vi "Six Motors Final.vi"() -> ()   [LabVIEW 2013]
uses:
  <vilib>/Analysis/Matrix/Datatypes/RealMatrix.ctl
  <vilib>/picture/3D Picture Control/Object/Create Object (drawable).vi
  <vilib>/picture/3D Picture Control/Object/Add Object (reference).vi
  <vilib>/Instr/_visa.llb/VISA Configure Serial Port (Instr).vi
  <vilib>/picture/3D Picture Control/NI_3D Picture Control.lvlib
  <vilib>/Analysis/Matrix/NI_Matrix.lvlib
panel:
  in  "Initial Values":bool
  out "x+y":dbl
  in  "Shoulder Angle":dbl=130.0
  in  "Pitch Exten":dbl
  in  "Elbow Angle":dbl=-130.0
  out "Input Palettes":string
  in  "Speed_PWM":i32(knob)=255 min=0 max=255 scale=0.0..255.0
  in  "Hard Home":bool
  in  "Pitch Closure":dbl(slide) min=0.0 max=130.0 scale=0.0..100.0
  out "FINAL TRANSFORMATION MATRIX":T1 format="%#.7f"
  in  "Base Angle":dbl
  in  "Pitch Roll":dbl
  in  "?":enum32{"Main Control", "Simulator"}(tab)
  out "Pitch Closure at Angle":i32
  out "Pitch Roll at Angle":i32
  out "Pitch Stretch at Angle":i32
  out "Elbow at Angle":i32
  out "Shoulder at Angle":i32
  out "Base at Angle":i16
  out "Position Palettes":string
  out "Error Palettes":string
  out "A Error":i32
  out "B Error":i32
  out "C Error":i32
  out "D Error":i32
  out "E Error":i32
  out "F Error":i32
  out "Serial Palettes":string
  out "Read Count":u32
  out "Write Count":u32
  in  "Home Position":bool
  out "Rhino Simulator":refnum<vi>(3d-picture)
  in  "Rhino Color":u32(colorbox)=11776947
  in  "Axis Color":u32(colorbox)
  in  "BackGround Color":u32(colorbox)=16777238
  in  "Alpha Value":dbl(slide)=0.47783251231527096 scale=0.0..1.0
  out "3D Picture 2":refnum<vi>(3d-picture)
  in  "STOP":bool
  in  "START":bool
  # "Close"
  # "Open"
  # "------------------------------------------------------- INSTRUCTIONS TO USE -------------------------------------------------------\n1 - This is a Rhino Simulator \n2 - Run the code and first select the Axis Color, Rhino Color , Background Color, Alpha Value and Object's Position w.r.t Rhino base\n3 - Press the Start Button. (At this point, you should be seeing a red cube, a rhino simulator and two axes, one moving and on non-moving).\n4 - Now change the angles of each joints (named with respect to the motors attached to them)\n5 - Get the values of angles which will eventually make the Rhino End Effector to move to the cubic object.\n6 - Now put these values in the orignal code and have fun! :) \n\nNote: At any point after pressing the Start button if either want to change the colors or object position, you will have to STOP the code and Run again."
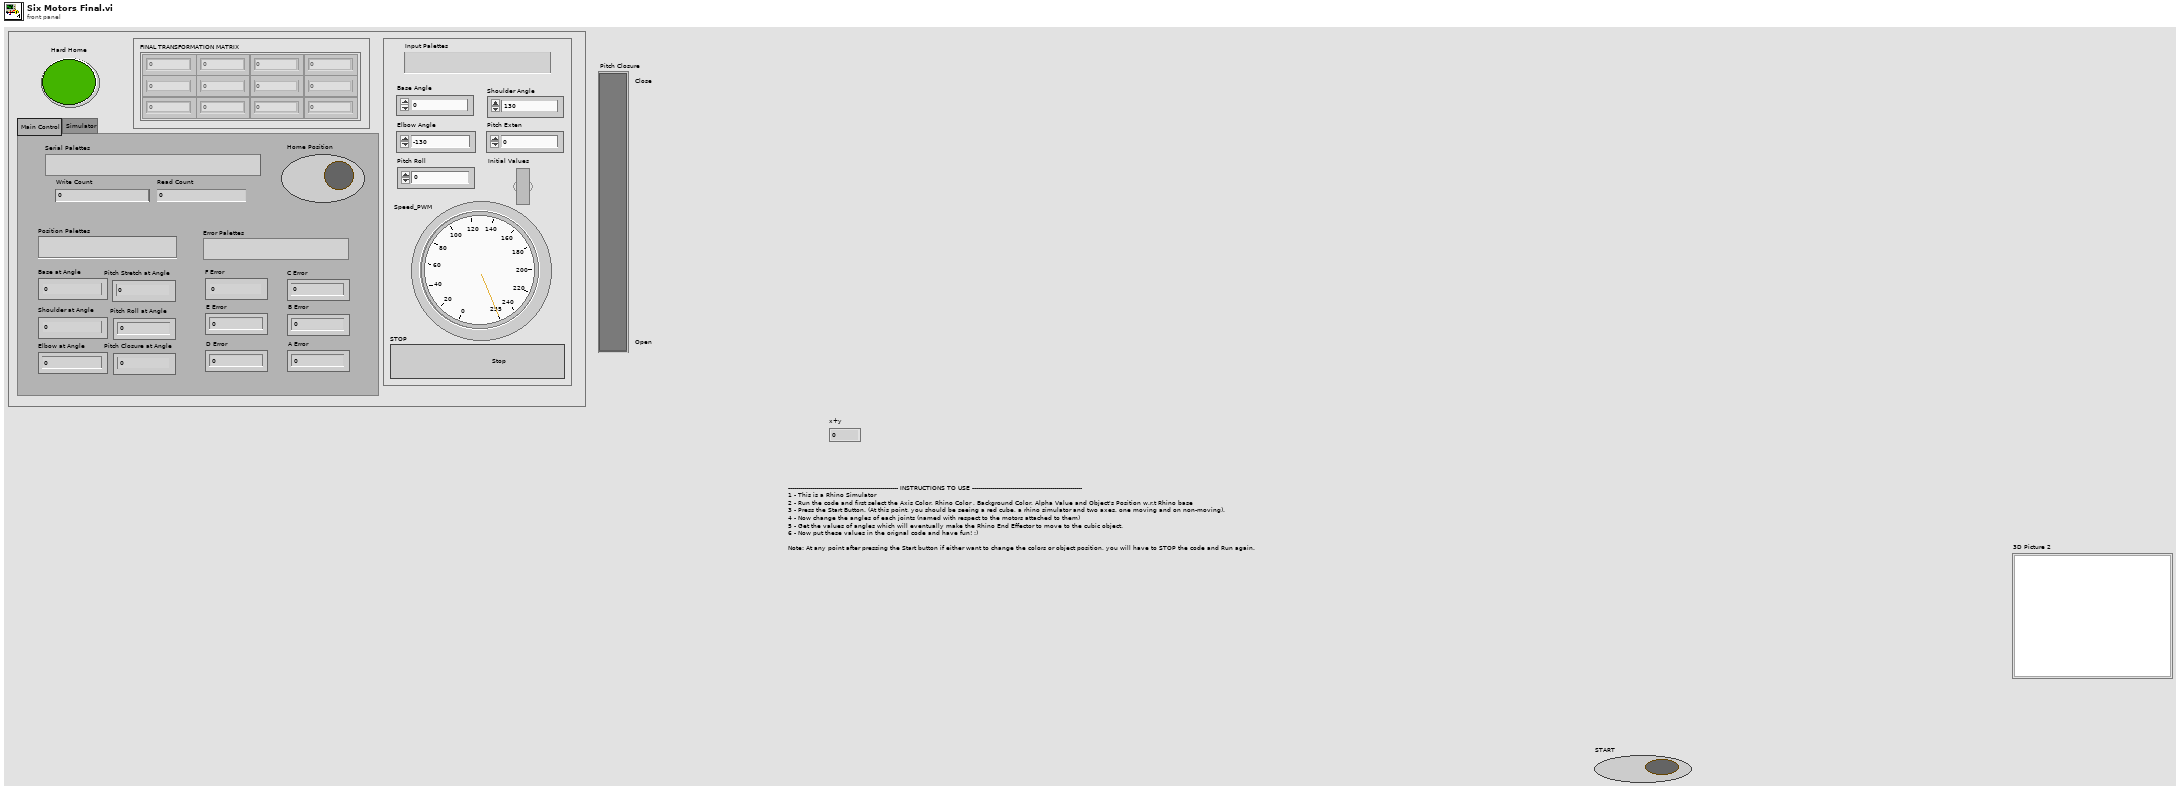
[diagram p1: front panel]
types:
  T1 = typedef "NI_Matrix.lvlib/RealMatrix.ctl" = dbl[][]
  T2 = cluster{"Red":sgl, "Green":sgl, "Blue":sgl, "Alpha":sgl}
  T3 = enum8{"Enabled", "Disabled", "Disabled and Grayed Out"}
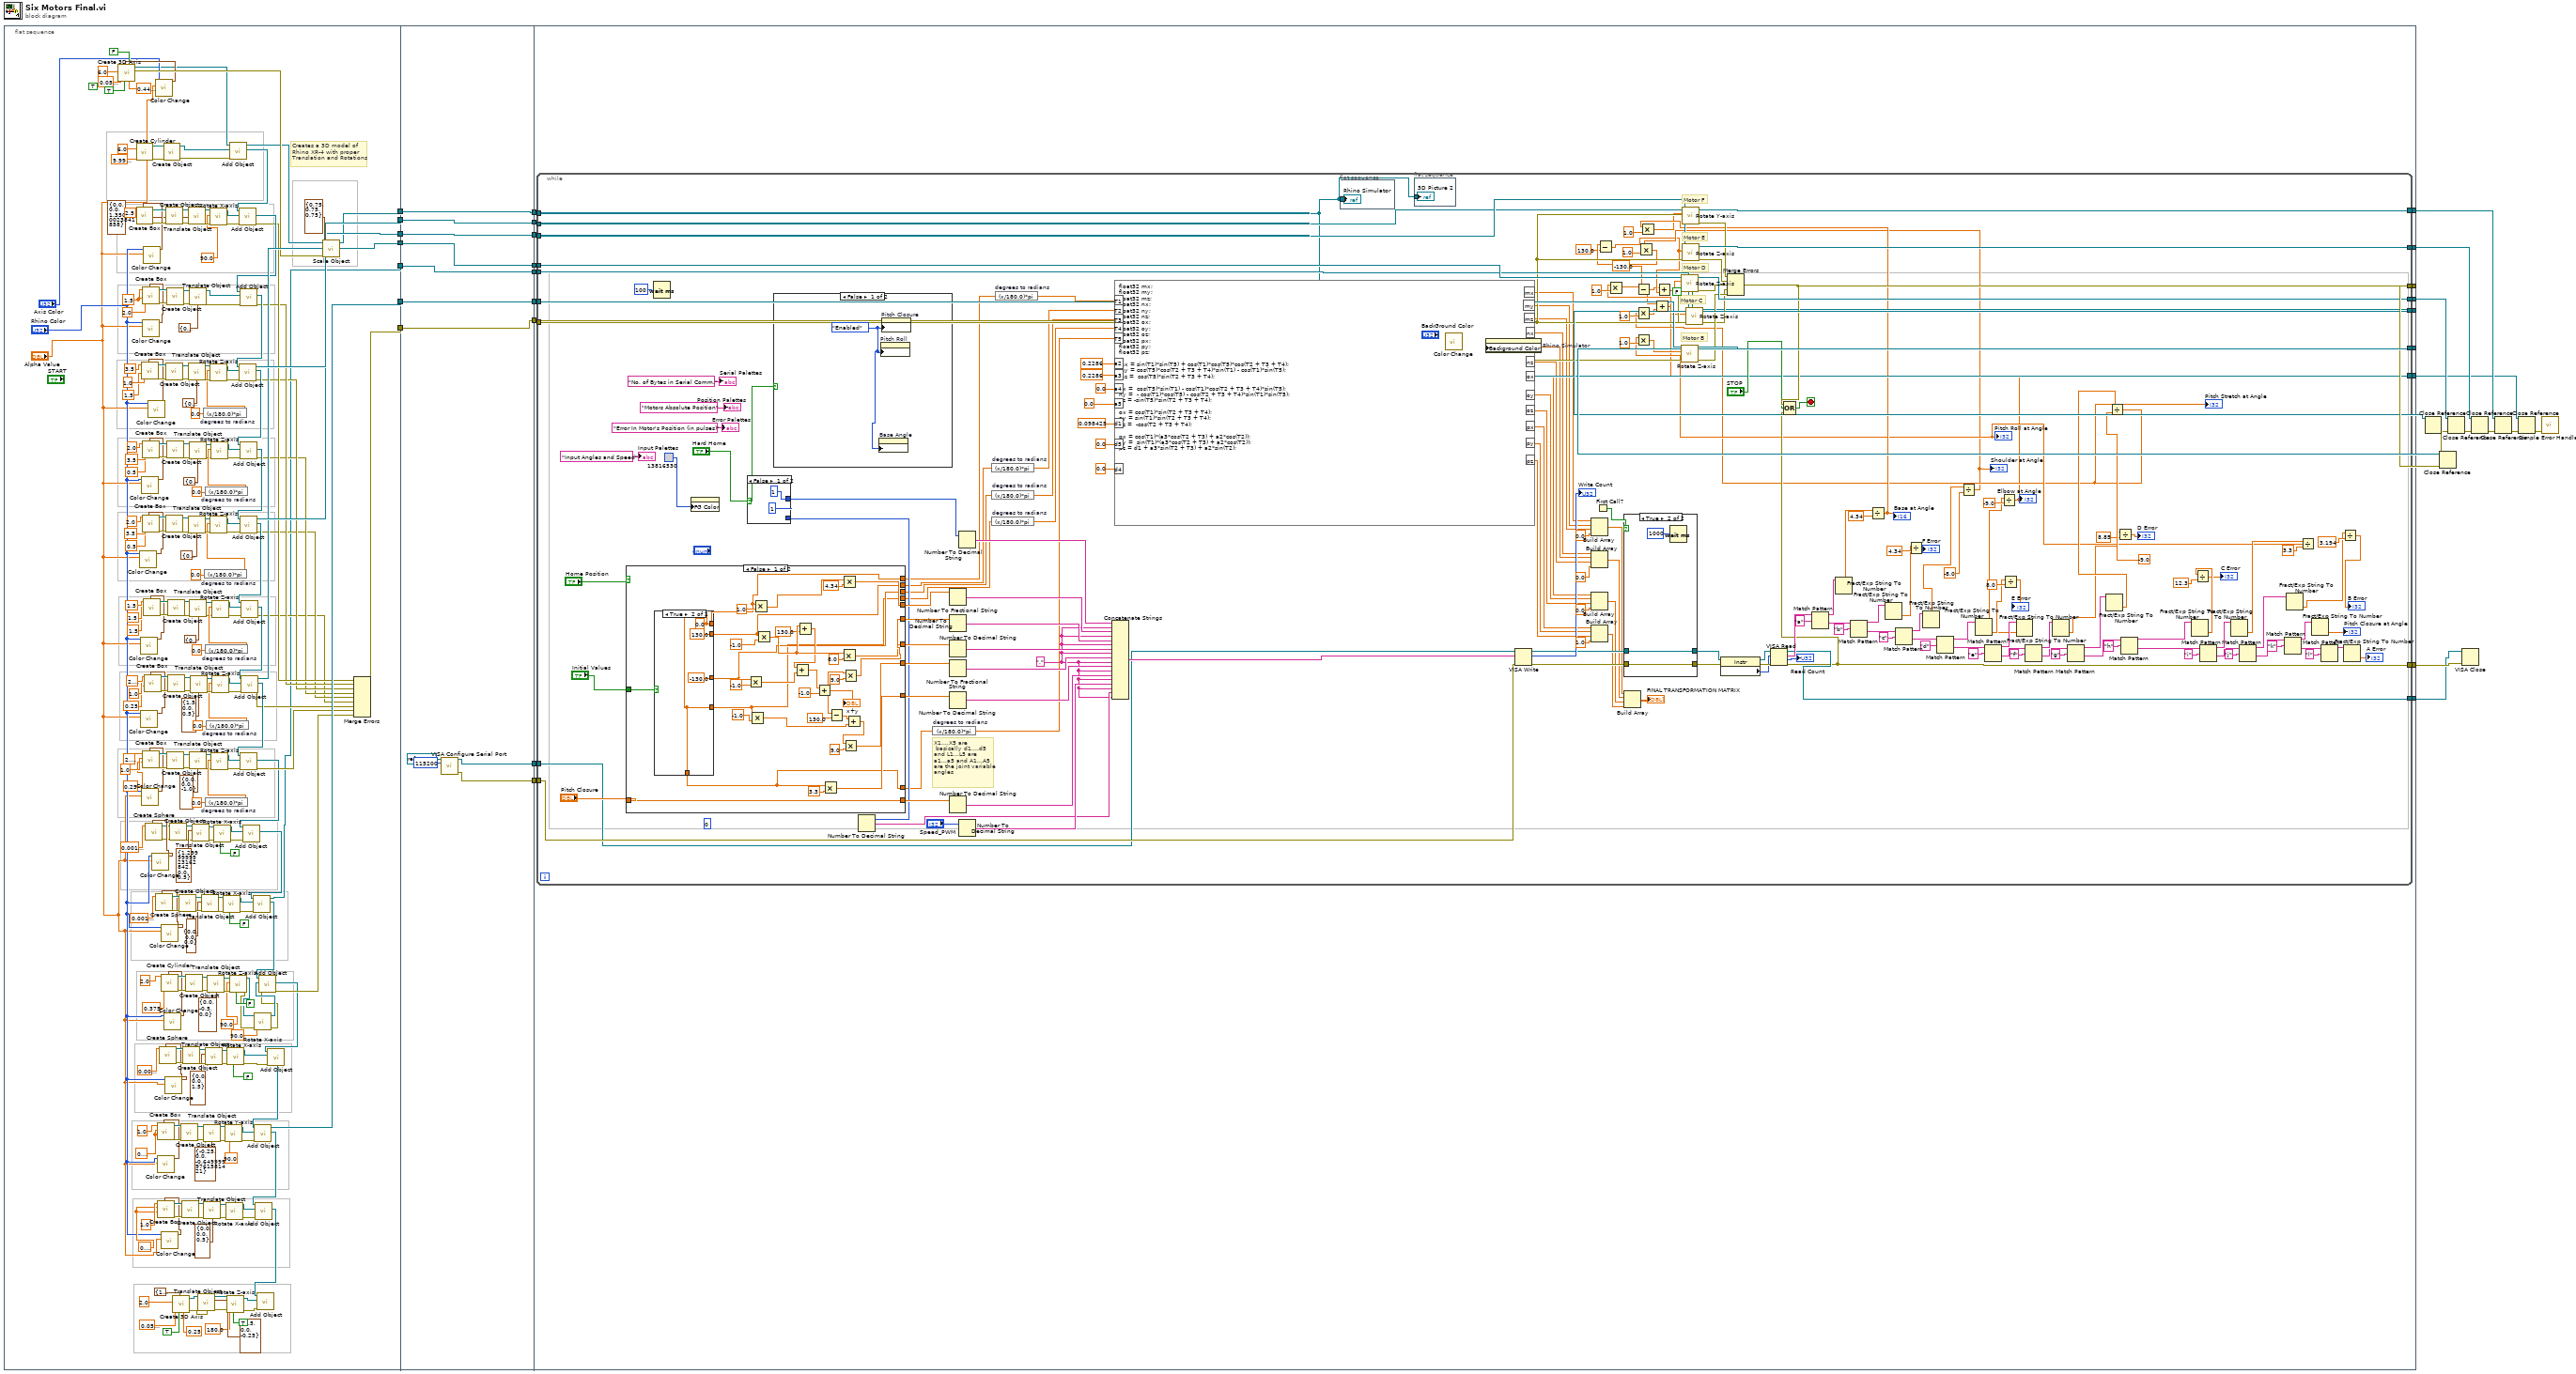
[diagram p0: block diagram]
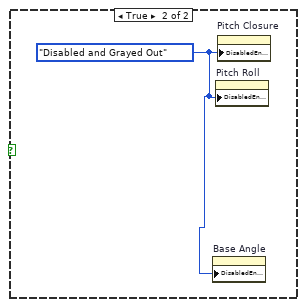
[diagram p2: hidden frame]
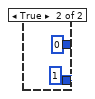
[diagram p3: hidden frame]
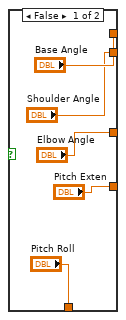
[diagram p4: hidden frame]
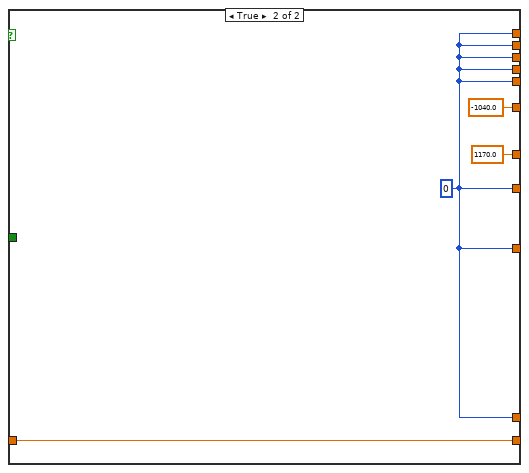
[diagram p5: hidden frame]
diagram:
  n1 = flat-sequence {
    tunnel: [w95] -> w31
    tunnel: [w285] -> w30
    tunnel: [w284] -> w29
    tunnel: [w283] -> w28
    tunnel: [w282] -> w27
    tunnel: [w38] -> w26
    tunnel: [w281] -> w25
    tunnel: [w296] -> w24
    tunnel: [w292] -> w23
    tunnel: [w290] -> w22
    tunnel: w31 -> [w296]
    tunnel: w30 -> [w295]
    tunnel: [w295] -> w21
    tunnel: w29 -> [w294]
    tunnel: [w294] -> w20
    tunnel: w28 -> [w293]
    tunnel: [w293] -> w19
    tunnel: w27 -> [w292]
    tunnel: w26 -> [w291]
    tunnel: [w291] -> w18
    tunnel: w25 -> [w290]
    tunnel: [w289] -> w4
    tunnel: [w288] -> w3
    tunnel: w24 -> [w314]
    tunnel: w23 -> [w310]
    tunnel: w22 -> [w311]
    tunnel: [w307] -> w13
    tunnel: [w306] -> w12
    tunnel: [w305] -> w11
    tunnel: [w304] -> w10
    tunnel: [w303] -> w9
    tunnel: [w302] -> w8
    tunnel: [w301] -> w6
    tunnel: w21 -> [w308]
    tunnel: w20 -> [w309]
    tunnel: w19 -> [w313]
    tunnel: w18 -> [w312]
    tunnel: w4 -> [w300]
    tunnel: w3 -> [w299]
    tunnel: [w298] -> w2
    tunnel: [w297] -> w1
    frame #0 {
      (unwired) TRUE ("Axis label?")
      w125 = sgl 0.1 ("Length Y")
      w127 = sgl 0.1 ("Length Y")
      w189 = sgl 1.5 ("Length X")
      w279 = sgl 2.5 ("Length X")
      # "Creates a 3D model of \nRhino XR-4 with proper \nTranslation and Rotations"
      n2 = call <vilib>:"Create Cylinder.vi"("Radius"=sgl 6.0, "Height"=sgl 0.0001) -> ("error out"=w77:errorcluster, "New Cylinder Refnum"=w78:refnum<vi>)  [unwired: 8 in]
      n3 = call <vilib>:"Color Change.vi"("Alpha"="Alpha Value", "Color"="Rhino Color") -> ("RGBA"=w115:cluster{"R":sgl, "G":sgl, "B":sgl, "A":sgl})  [unwired: 9 in]
      n4 = call <vilib>:"Color Change.vi"("Alpha"="Alpha Value", "Color"="Rhino Color") -> ("RGBA"=w116:cluster{"R":sgl, "G":sgl, "B":sgl, "A":sgl})  [unwired: 9 in]
      n5 = call <vilib>:"Color Change.vi"("Alpha"="Alpha Value", "Color"="Rhino Color") -> ("RGBA"=w117:cluster{"R":sgl, "G":sgl, "B":sgl, "A":sgl})  [unwired: 9 in]
      n6 = call <vilib>:"Color Change.vi"("Alpha"="Alpha Value", "Color"="Rhino Color") -> ("RGBA"=w113:cluster{"R":sgl, "G":sgl, "B":sgl, "A":sgl})  [unwired: 9 in]
      n7 = call <vilib>:"Color Change.vi"("Alpha"="Alpha Value", "Color"="Rhino Color") -> ("RGBA"=w118:cluster{"R":sgl, "G":sgl, "B":sgl, "A":sgl})  [unwired: 9 in]
      n8 = call <vilib>:"Create Box.vi"("Color"=w115, "Length Z"=sgl 0.5, "Length Y"=sgl 3.5, "Length X"=sgl 2.0) -> ("error out"=w234:errorcluster, "New Box Refnum"=w240:refnum<vi>)  [unwired: 6 in]
      n9 = call <vilib>:"Color Change.vi"("Alpha"="Alpha Value", "Color"="Rhino Color") -> ("RGBA"=w112:cluster{"R":sgl, "G":sgl, "B":sgl, "A":sgl})  [unwired: 9 in]
      n10 = call <vilib>:"Create Box.vi"("Color"=w112, "Length Z"=w189, "Length Y"=sgl 2.0, "Length X"=w189) -> ("error out"=w266:errorcluster, "New Box Refnum"=w263:refnum<vi>)  [unwired: 6 in]
      n11 = call <vilib>:"Create Box.vi"("Color"=w113, "Length Z"=sgl 0.5, "Length Y"=sgl 3.5, "Length X"=sgl 2.0) -> ("error out"=w247:errorcluster, "New Box Refnum"=w241:refnum<vi>)  [unwired: 6 in]
      n12 = call <vilib>:"Create Box.vi"("Color"=w118, "Length Z"=sgl 0.25 ("Length X"), "Length Y"=sgl 1.0 ("Length X"), "Length X"=sgl 2.7) -> ("error out"=w204:errorcluster, "New Box Refnum"=w198:refnum<vi>)  [unwired: 6 in]
      n13 = call <vilib>:"Color Change.vi"("Alpha"="Alpha Value", "Color"="Rhino Color") -> ("RGBA"=w123:cluster{"R":sgl, "G":sgl, "B":sgl, "A":sgl})  [unwired: 9 in]
      n14 = call <vilib>:"Create Box.vi"("Color"=w123, "Length Z"=w279, "Length Y"=w279, "Length X"=w279) -> ("error out"=w269:errorcluster, "New Box Refnum"=w280:refnum<vi>)  [unwired: 6 in]
      n15 = call <vilib>:"Create Box.vi"("Color"=w116, "Length Z"=sgl 1.5 ("Length X"), "Length Y"=sgl 1.5 ("Length X"), "Length X"=sgl 1.5) -> ("error out"=w226:errorcluster, "New Box Refnum"=w220:refnum<vi>)  [unwired: 6 in]
      n16 = call <vilib>:"Create Box.vi"("Color"=w117, "Length Z"=sgl 0.25 ("Length X"), "Length Y"=sgl 1.0 ("Length X"), "Length X"=sgl 2.7) -> ("error out"=w213:errorcluster, "New Box Refnum"=w219:refnum<vi>)  [unwired: 6 in]
      n17 = call <vilib>:"Color Change.vi"("Alpha"="Alpha Value", "Color"="Rhino Color") -> ("RGBA"=w114:cluster{"R":sgl, "G":sgl, "B":sgl, "A":sgl})  [unwired: 9 in]
      n18 = call <vilib>:"Create Box.vi"("Color"=w114, "Length Z"=sgl 1.5, "Length Y"=sgl 1.0, "Length X"=sgl 3.5) -> ("error out"=w256:errorcluster, "New Box Refnum"=w262:refnum<vi>)  [unwired: 6 in]
      n19 = call <vilib>:"Color Change.vi"("Alpha"="Alpha Value", "Color"="Rhino Color") -> ("RGBA"=w67:cluster{"R":sgl, "G":sgl, "B":sgl, "A":sgl})  [unwired: 9 in]
      n20 = call <vilib>:"Create Sphere.vi"("Color"=w67, "Radius"=sgl 0.001 ("Length X")) -> ("error out"=w59:errorcluster, "New Sphere Refnum"=w65:refnum<vi>)  [unwired: 8 in]
      n21 = call <vilib>:"Color Change.vi"("Alpha"="Alpha Value", "Color"="Axis Color") -> ("RGBA"=w111:cluster{"R":sgl, "G":sgl, "B":sgl, "A":sgl})  [unwired: 9 in]
      n22 = call <vilib>:"Create 3D Axis.vi"("Character Size"=sgl 0.45, "Half plane?"=FALSE, "Axis label?"=TRUE, "Color"=w111, "Radius"=sgl 0.05, "Length"=sgl 6.0) -> ("error out"=w161:errorcluster, "New Object Refnum"=w75:refnum<vi>)  [unwired: 4 in]
      n23 = call <vilib>:"Color Change.vi"("Alpha"="Alpha Value", "Color"="Rhino Color") -> ("RGBA"=w120:cluster{"R":sgl, "G":sgl, "B":sgl, "A":sgl})  [unwired: 9 in]
      n24 = call <vilib>:"Create Box.vi"("Color"=w120, "Length Z"=w127, "Length Y"=w127, "Length X"=sgl 1.0) -> ("error out"=w145:errorcluster, "New Box Refnum"=w139:refnum<vi>)  [unwired: 6 in]
      n25 = call <vilib>:"Color Change.vi"("Alpha"="Alpha Value", "Color"="Rhino Color") -> ("RGBA"=w121:cluster{"R":sgl, "G":sgl, "B":sgl, "A":sgl})  [unwired: 9 in]
      n26 = call <vilib>:"Create Box.vi"("Color"=w121, "Length Z"=w125, "Length Y"=w125, "Length X"=sgl 1.0) -> ("error out"=w132:errorcluster, "New Box Refnum"=w138:refnum<vi>)  [unwired: 6 in]
      n27 = call <vilib>:"Color Change.vi"("Alpha"="Alpha Value", "Color"="Rhino Color") -> ("RGBA"=w43:cluster{"R":sgl, "G":sgl, "B":sgl, "A":sgl})  [unwired: 9 in]
      n28 = call <vilib>:"Create Sphere.vi"("Color"=w43, "Radius"=sgl 0.001 ("Length X")) -> ("error out"=w51:errorcluster, "New Sphere Refnum"=w45:refnum<vi>)  [unwired: 8 in]
      n29 = call-poly <vilib>:"Create Object.vi"("error in (no error)"=w77, "Geometry"=w78) -> ("error out"=w33:errorcluster, "Scene:New Object"=w34:refnum<vi>)  [unwired: 8 in]
      n30 = call <vilib>:"Color Change.vi"("Alpha"="Alpha Value", "Color"="Rhino Color") -> ("RGBA"=w119:cluster{"R":sgl, "G":sgl, "B":sgl, "A":sgl})  [unwired: 9 in]
      n31 = call <vilib>:"Create Cylinder.vi"("Color"=w119, "Radius"=sgl 0.375, "Height"=sgl 2.0) -> ("error out"=w193:errorcluster, "New Cylinder Refnum"=w197:refnum<vi>)  [unwired: 7 in]
      n32 = call <vilib>:"Color Change.vi"("Alpha"="Alpha Value", "Color"="Rhino Color") -> ("RGBA"=w98:cluster{"R":sgl, "G":sgl, "B":sgl, "A":sgl})  [unwired: 9 in]
      n33 = call <vilib>:"Create Sphere.vi"("Color"=w98, "Radius"=sgl 0.01 ("Length X")) -> ("error out"=w106:errorcluster, "New Sphere Refnum"=w100:refnum<vi>)  [unwired: 8 in]
      n34 = call-poly <vilib>:"Create Object.vi"("error in (no error)"=w269, "Geometry"=w280) -> ("error out"=w270:errorcluster, "Scene:New Object"=w274:refnum<vi>)  [unwired: 8 in]
      n35 = call-poly <vilib>:"Create Object.vi"("error in (no error)"=w256, "Geometry"=w262) -> ("error out"=w257:errorcluster, "Scene:New Object"=w261:refnum<vi>)  [unwired: 8 in]
      n36 = call-poly <vilib>:"Create Object.vi"("error in (no error)"=w234, "Geometry"=w240) -> ("error out"=w235:errorcluster, "Scene:New Object"=w239:refnum<vi>)  [unwired: 8 in]
      n37 = call-poly <vilib>:"Create Object.vi"("error in (no error)"=w266, "Geometry"=w263) -> ("error out"=w265:errorcluster, "Scene:New Object"=w264:refnum<vi>)  [unwired: 8 in]
      n38 = call-poly <vilib>:"Create Object.vi"("error in (no error)"=w247, "Geometry"=w241) -> ("error out"=w246:errorcluster, "Scene:New Object"=w242:refnum<vi>)  [unwired: 8 in]
      n39 = call-poly <vilib>:"Create Object.vi"("error in (no error)"=w204, "Geometry"=w198) -> ("error out"=w203:errorcluster, "Scene:New Object"=w199:refnum<vi>)  [unwired: 8 in]
      n40 = call-poly <vilib>:"Create Object.vi"("error in (no error)"=w226, "Geometry"=w220) -> ("error out"=w225:errorcluster, "Scene:New Object"=w221:refnum<vi>)  [unwired: 8 in]
      n41 = call-poly <vilib>:"Create Object.vi"("error in (no error)"=w213, "Geometry"=w219) -> ("error out"=w214:errorcluster, "Scene:New Object"=w218:refnum<vi>)  [unwired: 8 in]
      n42 = call-poly <vilib>:"Create Object.vi"("error in (no error)"=w59, "Geometry"=w65) -> ("error out"=w60:errorcluster, "Scene:New Object"=w64:refnum<vi>)  [unwired: 8 in]
      n43 = call <vilib>:"Create 3D Axis.vi"("Character Size"=sgl 0.25, "Axis label?"=TRUE, "Color"=T2 {"Red"=1.0, "Green"=0.0, "Blue"=1.0, "Alpha"=1.0}, "Radius"=sgl 0.05, "Length"=sgl 2.0) -> ("error out"=w86:errorcluster, "New Object Refnum"=w87:refnum<vi>)  [unwired: 5 in]
      n44 = call-poly <vilib>:"Create Object.vi"("error in (no error)"=w51, "Geometry"=w45) -> ("error out"=w50:errorcluster, "Scene:New Object"=w46:refnum<vi>)  [unwired: 8 in]
      n45 = call-poly <vilib>:"Create Object.vi"("error in (no error)"=w145, "Geometry"=w139) -> ("error out"=w144:errorcluster, "Scene:New Object"=w140:refnum<vi>)  [unwired: 8 in]
      n46 = call-poly <vilib>:"Create Object.vi"("error in (no error)"=w132, "Geometry"=w138) -> ("error out"=w133:errorcluster, "Scene:New Object"=w137:refnum<vi>)  [unwired: 8 in]
      n47 = call-poly <vilib>:"Create Object.vi"("error in (no error)"=w106, "Geometry"=w100) -> ("error out"=w105:errorcluster, "Scene:New Object"=w101:refnum<vi>)  [unwired: 8 in]
      n48 = call-poly <vilib>:"Create Object.vi"("error in (no error)"=w193, "Geometry"=w197) -> ("error out"=w194:errorcluster, "Scene:New Object"=w196:refnum<vi>)  [unwired: 8 in]
      n49 = call <vilib>:"Translate Object.vi"("error in (no error)"=w270, "Translation"=cluster{"X":sgl, "Y":sgl, "Z":sgl} {"X"=0.0, "Y"=0.0, "Z"=1.35}, "Scene.Object In"=w274) -> ("error out"=w271:errorcluster, "Scene.Object Out"=w268:refnum<vi>)  [unwired: 7 in]
      n50 = call <vilib>:"Translate Object.vi"("error in (no error)"=w257, "Translation"=cluster{"X":sgl, "Y":sgl, "Z":sgl} {"X"=0.5, "Y"=1.0, "Z"=0.0}, "Scene.Object In"=w261) -> ("error out"=w258:errorcluster, "Scene.Object Out"=w255:refnum<vi>)  [unwired: 7 in]
      n51 = call <vilib>:"Translate Object.vi"("error in (no error)"=w235, "Translation"=cluster{"X":sgl, "Y":sgl, "Z":sgl} {"X"=0.0, "Y"=0.0, "Z"=-2.0}, "Scene.Object In"=w239) -> ("error out"=w236:errorcluster, "Scene.Object Out"=w233:refnum<vi>)  [unwired: 7 in]
      n52 = call <vilib>:"Translate Object.vi"("error in (no error)"=w265, "Translation"=cluster{"X":sgl, "Y":sgl, "Z":sgl} {"X"=0.0, "Y"=1.0, "Z"=0.0}, "Scene.Object In"=w264) -> ("error out"=w148:errorcluster, "Scene.Object Out"=w149:refnum<vi>)  [unwired: 7 in]
      n53 = call <vilib>:"Translate Object.vi"("error in (no error)"=w246, "Translation"=cluster{"X":sgl, "Y":sgl, "Z":sgl} {"X"=0.7, "Y"=1.3, "Z"=1.0}, "Scene.Object In"=w242) -> ("error out"=w245:errorcluster, "Scene.Object Out"=w248:refnum<vi>)  [unwired: 7 in]
      n54 = call <vilib>:"Translate Object.vi"("error in (no error)"=w203, "Translation"=cluster{"X":sgl, "Y":sgl, "Z":sgl} {"X"=0.0, "Y"=0.0, "Z"=-1.0}, "Scene.Object In"=w199) -> ("error out"=w202:errorcluster, "Scene.Object Out"=w205:refnum<vi>)  [unwired: 7 in]
      n55 = call <vilib>:"Translate Object.vi"("error in (no error)"=w225, "Translation"=cluster{"X":sgl, "Y":sgl, "Z":sgl} {"X"=0.0, "Y"=1.8, "Z"=1.0}, "Scene.Object In"=w221) -> ("error out"=w224:errorcluster, "Scene.Object Out"=w227:refnum<vi>)  [unwired: 7 in]
      n56 = call <vilib>:"Translate Object.vi"("error in (no error)"=w214, "Translation"=cluster{"X":sgl, "Y":sgl, "Z":sgl} {"X"=1.5, "Y"=0.0, "Z"=0.5}, "Scene.Object In"=w218) -> ("error out"=w215:errorcluster, "Scene.Object Out"=w212:refnum<vi>)  [unwired: 7 in]
      n57 = call <vilib>:"Translate Object.vi"("error in (no error)"=w60, "Translation"=cluster{"X":sgl, "Y":sgl, "Z":sgl} {"X"=1.3, "Y"=0.0, "Z"=0.5}, "Scene.Object In"=w64) -> ("error out"=w61:errorcluster, "Scene.Object Out"=w58:refnum<vi>)  [unwired: 7 in]
      n58 = call <vilib>:"Translate Object.vi"("error in (no error)"=w86, "Translation"=cluster{"X":sgl, "Y":sgl, "Z":sgl} {"X"=0.5, "Y"=0.0, "Z"=-0.25}, "Scene.Object In"=w87) -> ("error out"=w83:errorcluster, "Scene.Object Out"=w84:refnum<vi>)  [unwired: 7 in]
      n59 = call <vilib>:"Translate Object.vi"("error in (no error)"=w50, "Translation"=cluster{"X":sgl, "Y":sgl, "Z":sgl} {"X"=0.0, "Y"=0.0, "Z"=0.0}, "Scene.Object In"=w46) -> ("error out"=w49:errorcluster, "Scene.Object Out"=w52:refnum<vi>)  [unwired: 7 in]
      n60 = call <vilib>:"Translate Object.vi"("error in (no error)"=w144, "Translation"=cluster{"X":sgl, "Y":sgl, "Z":sgl} {"X"=-0.25, "Y"=0.0, "Z"=-0.65}, "Scene.Object In"=w140) -> ("error out"=w143:errorcluster, "Scene.Object Out"=w146:refnum<vi>)  [unwired: 7 in]
      n61 = expression code="(x/180.0)*pi" "degrees to radians"(0.0) -> (w253:dbl)
      n62 = call <vilib>:"Translate Object.vi"("error in (no error)"=w133, "Translation"=cluster{"X":sgl, "Y":sgl, "Z":sgl} {"X"=0.0, "Y"=0.0, "Z"=0.5}, "Scene.Object In"=w137) -> ("error out"=w134:errorcluster, "Scene.Object Out"=w131:refnum<vi>)  [unwired: 7 in]
      n63 = expression code="(x/180.0)*pi" "degrees to radians"(0.0) -> (w231:dbl)
      n64 = expression code="(x/180.0)*pi" "degrees to radians"(0.0) -> (w250:dbl)
      n65 = expression code="(x/180.0)*pi" "degrees to radians"(0.0) -> (w207:dbl)
      n66 = expression code="(x/180.0)*pi" "degrees to radians"(0.0) -> (w228:dbl)
      n67 = call <vilib>:"Translate Object.vi"("error in (no error)"=w105, "Translation"=cluster{"X":sgl, "Y":sgl, "Z":sgl} {"X"=0.0, "Y"=0.0, "Z"=1.5}, "Scene.Object In"=w101) -> ("error out"=w104:errorcluster, "Scene.Object Out"=w107:refnum<vi>)  [unwired: 7 in]
      n68 = expression code="(x/180.0)*pi" "degrees to radians"(0.0) -> (w210:dbl)
      n69 = call <vilib>:"Translate Object.vi"("error in (no error)"=w194, "Translation"=cluster{"X":sgl, "Y":sgl, "Z":sgl} {"X"=0.0, "Y"=-0.5, "Z"=0.0}, "Scene.Object In"=w196) -> ("error out"=w195:errorcluster, "Scene.Object Out"=w192:refnum<vi>)  [unwired: 7 in]
      n70 = call <vilib>:"Rotate X-axis.vi"("error in (no error)"=w271, "angle"=90.0, "Scene Object In"=w268) -> ("error out"=w273:errorcluster, "Scene Object Out"=w272:refnum<vi>)  [unwired: 7 in]
      n71 = call <vilib>:"Rotate Z-axis.vi"("error in (no error)"=w258, "angle"=w253, "Scene Object In"=w255) -> ("error out"=w260:errorcluster, "Scene Object Out"=w259:refnum<vi>)  [unwired: 7 in]
      n72 = call <vilib>:"Rotate Z-axis.vi"("error in (no error)"=w236, "angle"=w231, "Scene Object In"=w233) -> ("error out"=w238:errorcluster, "Scene Object Out"=w237:refnum<vi>)  [unwired: 7 in]
      n73 = call <vilib>:"Rotate Z-axis.vi"("error in (no error)"=w245, "angle"=w250, "Scene Object In"=w248) -> ("error out"=w243:errorcluster, "Scene Object Out"=w244:refnum<vi>)  [unwired: 7 in]
      n74 = call <vilib>:"Rotate Z-axis.vi"("error in (no error)"=w202, "angle"=w207, "Scene Object In"=w205) -> ("error out"=w200:errorcluster, "Scene Object Out"=w201:refnum<vi>)  [unwired: 7 in]
      n75 = call <vilib>:"Rotate Z-axis.vi"("error in (no error)"=w224, "angle"=w228, "Scene Object In"=w227) -> ("error out"=w222:errorcluster, "Scene Object Out"=w223:refnum<vi>)  [unwired: 7 in]
      n76 = call <vilib>:"Rotate Z-axis.vi"("error in (no error)"=w215, "angle"=w210, "Scene Object In"=w212) -> ("error out"=w217:errorcluster, "Scene Object Out"=w216:refnum<vi>)  [unwired: 7 in]
      n77 = call <vilib>:"Rotate X-axis.vi"("Relative?"=FALSE, "error in (no error)"=w61, "Scene Object In"=w58) -> ("error out"=w63:errorcluster, "Scene Object Out"=w62:refnum<vi>)  [unwired: 7 in]
      n78 = call <vilib>:"Rotate X-axis.vi"("Relative?"=FALSE, "error in (no error)"=w49, "Scene Object In"=w52) -> ("error out"=w47:errorcluster, "Scene Object Out"=w48:refnum<vi>)  [unwired: 7 in]
      n79 = call <vilib>:"Rotate Y-axis.vi"("error in (no error)"=w143, "angle"=90.0, "Scene Object In"=w146) -> ("error out"=w141:errorcluster, "Scene Object Out"=w142:refnum<vi>)  [unwired: 7 in]
      n80 = call <vilib>:"Rotate X-axis.vi"("error in (no error)"=w134, "Scene Object In"=w131) -> ("error out"=w136:errorcluster, "Scene Object Out"=w135:refnum<vi>)  [unwired: 8 in]
      n81 = call <vilib>:"Rotate Z-axis.vi"("Relative?"=TRUE, "error in (no error)"=w83, "angle"=sgl 180.0, "Scene Object In"=w84) -> ("error out"=w82:errorcluster, "Scene Object Out"=w81:refnum<vi>)  [unwired: 6 in]
      n82 = call <vilib>:"Rotate X-axis.vi"("Relative?"=FALSE, "error in (no error)"=w104, "Scene Object In"=w107) -> ("error out"=w102:errorcluster, "Scene Object Out"=w103:refnum<vi>)  [unwired: 7 in]
      n83 = call-poly <vilib>:"Add Object.vi"("error in (no error)"=w33, "New Object In"=w34, "Scene Object In"=w75) -> ("New Object Out"=w76:refnum<vi>, "Scene Object Out"=w74:refnum<vi>)  [unwired: 6 in, 1 out]
      n84 = call <vilib>:"Rotate Z-axis.vi"("Relative?"=FALSE, "error in (no error)"=w195, "angle"=90.0, "Scene Object In"=w192) -> ("error out"=w70:errorcluster, "Scene Object Out"=w72:refnum<vi>)  [unwired: 6 in]
      n85 = call-poly <vilib>:"Add Object.vi"("error in (no error)"=w273, "New Object In"=w272, "Scene Object In"=w76) -> ("error out"=w160:errorcluster, "New Object Out"=w169:refnum<vi>)  [unwired: 6 in, 1 out]
      n86 = call-poly <vilib>:"Add Object.vi"("error in (no error)"=w148, "New Object In"=w149, "Scene Object In"=w169) -> ("error out"=w159:errorcluster, "New Object Out"=w168:refnum<vi>)  [unwired: 6 in, 1 out]
      n87 = call-poly <vilib>:"Add Object.vi"("error in (no error)"=w260, "New Object In"=w259, "Scene Object In"=w168) -> ("error out"=w158:errorcluster, "New Object Out"=w167:refnum<vi>, "Scene Object Out"=w285:refnum<vi>)  [unwired: 6 in]
      n88 = call-poly <vilib>:"Add Object.vi"("error in (no error)"=w243, "New Object In"=w244, "Scene Object In"=w167) -> ("error out"=w157:errorcluster, "New Object Out"=w166:refnum<vi>)  [unwired: 6 in, 1 out]
      n89 = call-poly <vilib>:"Add Object.vi"("error in (no error)"=w238, "New Object In"=w237, "Scene Object In"=w166) -> ("error out"=w156:errorcluster, "New Object Out"=w165:refnum<vi>, "Scene Object Out"=w284:refnum<vi>)  [unwired: 6 in]
      n90 = call-poly <vilib>:"Add Object.vi"("error in (no error)"=w222, "New Object In"=w223, "Scene Object In"=w165) -> ("error out"=w155:errorcluster, "New Object Out"=w164:refnum<vi>)  [unwired: 6 in, 1 out]
      n91 = call-poly <vilib>:"Add Object.vi"("error in (no error)"=w217, "New Object In"=w216, "Scene Object In"=w164) -> ("error out"=w154:errorcluster, "New Object Out"=w163:refnum<vi>, "Scene Object Out"=w283:refnum<vi>)  [unwired: 6 in]
      n92 = call-poly <vilib>:"Add Object.vi"("error in (no error)"=w200, "New Object In"=w201, "Scene Object In"=w163) -> ("error out"=w153:errorcluster, "New Object Out"=w55:refnum<vi>)  [unwired: 6 in, 1 out]
      n93 = call-poly <vilib>:"Add Object.vi"("error in (no error)"=w63, "New Object In"=w62, "Scene Object In"=w55) -> ("New Object Out"=w42:refnum<vi>)  [unwired: 6 in, 2 out]
      n94 = call-poly <vilib>:"Add Object.vi"("error in (no error)"=w47, "New Object In"=w48, "Scene Object In"=w42) -> ("New Object Out"=w41:refnum<vi>, "Scene Object Out"=w38:refnum<vi>)  [unwired: 6 in, 1 out]
      n95 = call <vilib>:"Rotate X-axis.vi"("error in (no error)"=w70, "angle"=90.0, "Scene Object In"=w72) -> ("error out"=w69:errorcluster, "Scene Object Out"=w71:refnum<vi>)  [unwired: 7 in]
      n96 = call-poly <vilib>:"Add Object.vi"("error in (no error)"=w69, "New Object In"=w71, "Scene Object In"=w41) -> ("error out"=w152:errorcluster, "New Object Out"=w32:refnum<vi>)  [unwired: 6 in, 1 out]
      n97 = call-poly <vilib>:"Add Object.vi"("error in (no error)"=w102, "New Object In"=w103, "Scene Object In"=w32) -> ("New Object Out"=w97:refnum<vi>)  [unwired: 6 in, 2 out]
      n98 = call-poly <vilib>:"Add Object.vi"("error in (no error)"=w141, "New Object In"=w142, "Scene Object In"=w97) -> ("New Object Out"=w129:refnum<vi>, "Scene Object Out"=w281:refnum<vi>)  [unwired: 6 in, 1 out]
      n99 = call-poly <vilib>:"Add Object.vi"("error in (no error)"=w136, "New Object In"=w135, "Scene Object In"=w129) -> ("New Object Out"=w93:refnum<vi>)  [unwired: 6 in, 2 out]
      n100 = call-poly <vilib>:"Add Object.vi"("error in (no error)"=w82, "New Object In"=w81, "Scene Object In"=w93) -> ()  [unwired: 6 in, 3 out]
      n101 = call <vilib>:"Scale Object.vi"("error in (no error)"=w161, "Scale"=cluster{"X":sgl, "Y":sgl, "Z":sgl} {"X"=0.75, "Y"=0.75, "Z"=0.75}, "Scene.Object In"=w74) -> ("Scene.Object Out"=w95:refnum<vi>)  [unwired: 7 in, 1 out]
      n102 = Merge Errors(w160, w159, w158, w157, w156, w155, w154, w153, w152) -> (w282:errorcluster)
    }
    frame #1 {
      n103 = call-poly "VISA Configure Serial Port"("VISA resource name"=refnum<visa-resource-name> "COM12", "baud rate (9600)"=u32 115200) -> ("VISA resource name out"=w289:refnum<visa-resource-name>, "error out"=w288:errorcluster)  [unwired: 12 in]
    }
    frame #2 {
      n104 = while {
        tunnel: w314 -> [w486]
        tunnel: w313 -> [w503]
        tunnel: w312 -> [w502]
        tunnel: w311 -> [w501]
        tunnel: w310 -> [w498]
        tunnel: w309 -> [w500]
        tunnel: w308 -> [w499]
        tunnel: [w497] -> w307
        tunnel: [w489] -> w306
        tunnel: [w481] -> w305
        tunnel: [w496] -> w304
        tunnel: [w495] -> w303
        tunnel: [w494] -> w302
        tunnel: [w486] -> w301
        tunnel: w300 -> [w369]
        tunnel: w299 -> [w370]
        tunnel: [w342] -> w298
        tunnel: [w368] -> w297
        stop <- w488 stop-if-true
        (unwired) u32 0 ("y")
        w376 = "," ("string")
        # "X1....X5 are\n basically d1....d5\nand L1...L5 are \na1...a5 and A1...A5\nare the joint variable\nangles"
        # "Motor B"
        # "Motor C"
        # "Motor D"
        # "Motor E"
        # "Motor F"
        n105 = case shown="False" "Home Position" {
          tunnel: [w541 w553] -> w448
          tunnel: [w516 -1040.0] -> w452
          tunnel: [w529 1170.0] -> w451
          tunnel: [w528 w553] -> w447
          tunnel: [w540 w553] -> w446
          tunnel: [w538 w554] -> w445
          tunnel: [w515 w553] -> w320
          tunnel: [w514 w553] -> w319
          tunnel: [w513 w553] -> w318
          tunnel: [w512 w553] -> w317
          tunnel: [w511 w553] -> w316
          tunnel: "Pitch Closure" -> [w538 w554]
          tunnel: "Initial Values" -> [w510 _]
          frame False {
            n106 = case shown="True" w510 {
              tunnel: ["Base Angle" w548] -> w515
              tunnel: ["Shoulder Angle" 130.0 ("Shoulder Angle")] -> w514
              tunnel: ["Elbow Angle" -130.0 ("Elbow Angle")] -> w513
              tunnel: ["Pitch Exten" w548] -> w512
              tunnel: ["Pitch Roll" w548] -> w511
              frame False {
              }
              frame True {
                w548 = 0.0 ("Base Angle")
              }
            }
            n107 = Multiply(x=w513, y=-1.0) -> (x*y=w518:dbl)
            n108 = Multiply(x=w512, y=-1.0) -> (x*y=w517:dbl)
            n109 = Multiply(x=w515, y=1.0) -> (x*y=w536:dbl)
            n110 = Multiply(x=w514, y=-1.0) -> (x*y=w527:dbl)
            n111 = Add(x=w527, y=130.0) -> (x+y=w525:dbl)
            n112 = Add(x=w525, y=w518) -> (x+y=w524:dbl)
            n113 = Add(x=w524, y=-1.0) -> (x+y=w522:dbl)
            "x+y" <- w522
            n114 = Multiply(x=w511, y=3.3) -> (x*y=w540:dbl)
            n115 = Subtract(x=w522, y=130.0) -> (x-y=w520:dbl)
            n116 = Multiply(x=w527, y=8.0) -> (x*y=w516:dbl)
            n117 = Multiply(x=w536, y=4.34) -> (x*y=w541:dbl)
            n118 = Multiply(x=w522, y=9.0) -> (x*y=w529:dbl)
            n119 = Add(x=w520, y=w517) -> (x+y=w519:dbl)
            n120 = Multiply(x=w519, y=9.0) -> (x*y=w528:dbl)
          }
          frame True {
            w553 = 0 ("F Want at position")
          }
        }
        n121 = Wait (ms)(milliseconds to wait=u32 100) -> ()  [unwired: 1 out]
        n122 = property class="TabCtl (strict)"("FG Color"=u32 13816530) -> ()  [unwired: 2 in, 2 out]
        n123 = case shown="False" "Hard Home" {
          tunnel: [1 ("number") 0 ("number")] -> w381
          tunnel: [1 ("number") 1 ("number")] -> w379
          frame False {
          }
          frame True {
          }
        }
        n124 = case shown="False" "Hard Home" {
          frame False {
            w504 = T3."Enabled" ("Disabled")
            n125 = property on="Base Angle" class="DigNum (strict)"("DisabledEnum"=w504) -> ()  [unwired: 2 in, 2 out]
            n126 = property on="Pitch Roll" class="DigNum (strict)"("DisabledEnum"=w504) -> ()  [unwired: 2 in, 2 out]
            n127 = property on="Pitch Closure" class="Slide (strict)"("DisabledEnum"=w504) -> ()  [unwired: 2 in, 2 out]
          }
          frame True {
            w505 = T3."Disabled and Grayed Out" ("Disabled")
            n128 = property on="Base Angle" class="DigNum (strict)"("DisabledEnum"=w505) -> ()  [unwired: 2 in, 2 out]
            n129 = property on="Pitch Roll" class="DigNum (strict)"("DisabledEnum"=w505) -> ()  [unwired: 2 in, 2 out]
            n130 = property on="Pitch Closure" class="Slide (strict)"("DisabledEnum"=w505) -> ()  [unwired: 2 in, 2 out]
          }
        }
        n131 = Number To Decimal String(number=w379) -> (decimal integer string=w377:string)  [unwired: 1 in]
        n132 = expression code="(x/180.0)*pi" "degrees to radians"(w316) -> (w384:dbl)
        n133 = Number To Fractional String(number=w448) -> (F-format string=w473:string)  [unwired: 3 in]
        n134 = Number To Decimal String(number=w452) -> (decimal integer string=w466:string)  [unwired: 1 in]
        n135 = Number To Decimal String(number=w451) -> (decimal integer string=w465:string)  [unwired: 1 in]
        n136 = Number To Fractional String(number=w447) -> (F-format string=w444:string)  [unwired: 3 in]
        n137 = Number To Decimal String(number=w446) -> (decimal integer string=w443:string)  [unwired: 1 in]
        n138 = Number To Decimal String(number=w445) -> (decimal integer string=w442:string)  [unwired: 1 in]
        n139 = Number To Decimal String(number=w381) -> (decimal integer string=w449:string)  [unwired: 1 in]
        n140 = Number To Decimal String(number="Speed_PWM") -> (decimal integer string=w441:string)  [unwired: 1 in]
        n141 = expression code="(x/180.0)*pi" "degrees to radians"(w319) -> (w387:dbl)
        n142 = expression code="(x/180.0)*pi" "degrees to radians"(w318) -> (w386:dbl)
        n143 = expression code="(x/180.0)*pi" "degrees to radians"(w317) -> (w385:dbl)
        n144 = expression code="(x/180.0)*pi" "degrees to radians"(w320) -> (w388:dbl)
        n145 = Concatenate Strings(w449, w376, w473, w376, w466, w376, w465, w376, w444, w376, w443, w376, w442, w376, w441, w376, w377, w376) -> (w474:string)
        n146 = formula code="float32 mx;\nfloat32 my;\nfloat32 mz;\nfloat32 nx;\nfloat32 ny;\nfloat32 nz;\nfloat32 ox;\nfloat32 oy;\nfloat32 oz;\nfloat32 px;\nfloat32 py;\nfloat32 pz;\n\nmx = sin(T1)*sin(T5) + cos(T1)*cos(T5)*cos(T2 + T3 + T4);\nmy = cos(T5)*cos(T2 + T3 + T4)*sin(T1) - cos(T1)*sin(T5);\nmz =  cos(T5)*sin(T2 + T3 + T4);\n\nnx =  cos(T5)*sin(T1) - cos(T1)*cos(T2 + T3 + T4)*sin(T5);\nny =  - cos(T1)*cos(T5) - cos(T2 + T3 + T4)*sin(T1)*sin(T5);\nnz = -sin(T5)*sin(T2 + T3 + T4);\n\nox = cos(T1)*sin(T2 + T3 + T4);\noy = sin(T1)*sin(T2 + T3 + T4);\noz =  -cos(T2 + T3 + T4);\n\npx = cos(T1)*(a3*cos(T2 + T3) + a2*cos(T2));\npy =  sin(T1)*(a3*cos(T2 + T3) + a2*cos(T2));\npz = d1 + a3*sin(T2 + T3) + a2*sin(T2);"("T1"=w388, "T2"=w387, "T3"=w386, "T4"=w385, "T5"=w384, "a2"=0.2286 ("input variable"), "a3"=0.2286 ("input variable"), "a4"=0.0 ("input variable"), "a5"=0.0 ("input variable"), "d1"=0.098425 ("input variable"), "d5"=0.0 ("input variable"), "d4"=0.0 ("input variable")) -> ("mx"=w409:sgl, "my"=w408:sgl, "mz"=w407:sgl, "nx"=w405:sgl, "ny"=w404:sgl, "nz"=w403:sgl, "ox"=w401:sgl, "oy"=w400:sgl, "oz"=w399:sgl, "px"=w397:sgl, "py"=w396:sgl, "pz"=w395:sgl)
        n147 = flat-sequence {
          tunnel: w486 -> [w561]
          frame #0 {
            "Rhino Simulator" <- w561
          }
        }
        n148 = flat-sequence {
          tunnel: w486 -> [w560]
          frame #0 {
            "3D Picture 2" <- w560
          }
        }
        n149 = call <vilib>:"Color Change.vi"("Color"="BackGround Color") -> ("RGBA"=w485:cluster{"R":sgl, "G":sgl, "B":sgl, "A":sgl})  [unwired: 10 in]
        n150 = property on="Rhino Simulator" class="SceneGraphDisp (strict)"("Background Color"=w485) -> ()  [unwired: 2 in, 2 out]
        n151 = VISA Write(VISA resource name=w369, write buffer=w474, error in (no error)=w370) -> (VISA resource name out=w469:refnum<visa-resource-name>, return count=→"Write Count":u32, error out=w468:errorcluster)
        n152 = Build Array(w409, w408, w407, sgl 0.0 ("element")) -> (w393:sgl[])
        n153 = Build Array(w405, w404, w403, sgl 0.0 ("element")) -> (w392:sgl[])
        n154 = Build Array(w401, w400, w399, sgl 0.0 ("element")) -> (w391:sgl[])
        n155 = Build Array(w397, w396, w395, sgl 1.0 ("element")) -> (w390:sgl[])
        n156 = First Call?() -> (First Call?: T/F=w467:bool)
        n157 = case shown="True" w467 {
          tunnel: w469 -> [w556 w558]
          tunnel: w468 -> [w555 w557]
          tunnel: [w556 w558] -> w418
          tunnel: [w555 w557] -> w417
          frame False {
          }
          frame True {
            n158 = Wait (ms)(milliseconds to wait=u32 1000) -> ()  [unwired: 1 out]
          }
        }
        n159 = Build Array(w393, w392, w391, w390) -> (→"FINAL TRANSFORMATION MATRIX":T1)
        n160 = property class="Instr"(reference=w418, error in=w417) -> (reference out=w420:refnum<visa-resource-name>, error out=w419:errorcluster, "Serial Settings:Number of Bytes at Serial Port"=w416:u32)
        n161 = VISA Read(VISA resource name=w420, byte count=w416, error in (no error)=w419) -> (VISA resource name out=w368:refnum<visa-resource-name>, read buffer=w478:string, return count=→"Read Count":u32, error out=w342:errorcluster)
        n162 = Match Pattern(string=w478, regular expression="a") -> (before substring=w476:string, after substring=w472:string)  [unwired: 1 in, 2 out]
        n163 = Fract/Exp String To Number(string=w476) -> (number=w366:dbl)  [unwired: 3 in, 1 out]
        n164 = Match Pattern(string=w472, regular expression="b") -> (before substring=w470:string, after substring=w464:string)  [unwired: 1 in, 2 out]
        n165 = Divide(x=w366, y=4.34) -> (x/y=w341:dbl)
        "Base at Angle" <- w341
        n166 = Multiply(x=w341, y=1.0) -> (x*y=w339:dbl)
        n167 = call <vilib>:"Rotate Y-axis.vi"("error in (no error)"=w498, "angle"=w339, "Scene Object In"=w499) -> ("error out"=w493:errorcluster, "Scene Object Out"=w494:refnum<vi>)  [unwired: 7 in]
        n168 = Fract/Exp String To Number(string=w470) -> (number=w364:dbl)  [unwired: 3 in, 1 out]
        n169 = Match Pattern(string=w464, regular expression="c") -> (before substring=w456:string, after substring=w463:string)  [unwired: 1 in, 2 out]
        n170 = Divide(x=w364, y=4.34) -> (x/y=→"F Error":dbl)
        n171 = Fract/Exp String To Number(string=w456) -> (number=w360:dbl)  [unwired: 3 in, 1 out]
        n172 = Match Pattern(string=w463, regular expression="d") -> (before substring=w455:string, after substring=w462:string)  [unwired: 1 in, 2 out]
        n173 = Divide(x=w360, y=-8.0) -> (x/y=w330:dbl)
        "Shoulder at Angle" <- w330
        n174 = Multiply(x=w330, y=1.0) -> (x*y=w329:dbl)
        n175 = Subtract(x=w329, y=130.0) -> (x-y=w325:dbl)
        n176 = call <vilib>:"Rotate Z-axis.vi"("error in (no error)"=w498, "angle"=w325, "Scene Object In"=w500) -> ("error out"=w492:errorcluster, "Scene Object Out"=w495:refnum<vi>)  [unwired: 7 in]
        n177 = Fract/Exp String To Number(string=w455) -> (number=w359:dbl)  [unwired: 3 in, 1 out]
        n178 = Match Pattern(string=w462, regular expression="e") -> (before substring=w454:string, after substring=w461:string)  [unwired: 1 in, 2 out]
        n179 = Divide(x=w359, y=8.0) -> (x/y=→"E Error":dbl)
        n180 = Fract/Exp String To Number(string=w454) -> (number=w352:dbl)  [unwired: 3 in, 1 out]
        n181 = Divide(x=w352, y=-9.0) -> (x/y=w331:dbl)
        "Elbow at Angle" <- w331
        n182 = Multiply(x=w331, y=1.0) -> (x*y=w327:dbl)
        n183 = Subtract(x=w327, y=-130.0) -> (x-y=w322:dbl)
        n184 = Add(x=w322, y=w325) -> (x+y=w324:dbl)
        n185 = call <vilib>:"Rotate Z-axis.vi"("error in (no error)"=w498, "angle"=w324, "Scene Object In"=w503) -> ("error out"=w491:errorcluster, "Scene Object Out"=w496:refnum<vi>)  [unwired: 7 in]
        n186 = Match Pattern(string=w461, regular expression="f") -> (before substring=w453:string, after substring=w425:string)  [unwired: 1 in, 2 out]
        n187 = Fract/Exp String To Number(string=w453) -> (number=w355:dbl)  [unwired: 3 in, 1 out]
        n188 = Match Pattern(string=w425, regular expression="g") -> (before substring=w427:string, after substring=w428:string)  [unwired: 1 in, 2 out]
        n189 = Fract/Exp String To Number(string=w427) -> (number=w357:dbl)  [unwired: 3 in, 1 out]
        n190 = Divide(x=w357, y=-9.0) -> (x/y=w332:dbl)
        "Pitch Stretch at Angle" <- w332
        n191 = Multiply(x=w332, y=1.0) -> (x*y=w323:dbl)
        n192 = Add(x=w322, y=w323) -> (x+y=w321:dbl)
        n193 = call <vilib>:"Rotate Z-axis.vi"("Relative?"=FALSE, "error in (no error)"=w498, "angle"=w321, "Scene Object In"=w502) -> ("error out"=w482:errorcluster, "Scene Object Out"=w481:refnum<vi>)  [unwired: 6 in]
        n194 = Divide(x=w355, y=8.85) -> (x/y=→"D Error":dbl)
        n195 = Match Pattern(string=w428, regular expression="h") -> (before substring=w430:string, after substring=w431:string)  [unwired: 1 in, 2 out]
        n196 = Fract/Exp String To Number(string=w430) -> (number=w349:dbl)  [unwired: 3 in, 1 out]
        n197 = Divide(x=w349, y=12.3) -> (x/y=→"C Error":dbl)
        n198 = Match Pattern(string=w431, regular expression="i") -> (before substring=w436:string, after substring=w432:string)  [unwired: 1 in, 2 out]
        n199 = Fract/Exp String To Number(string=w436) -> (number=w346:dbl)  [unwired: 3 in, 1 out]
        n200 = Match Pattern(string=w432, regular expression="j") -> (before substring=w437:string, after substring=w433:string)  [unwired: 1 in, 2 out]
        n201 = Match Pattern(string=w433, regular expression="k") -> (before substring=w438:string, after substring=w422:string)  [unwired: 1 in, 2 out]
        n202 = Fract/Exp String To Number(string=w437) -> (number=w344:dbl)  [unwired: 3 in, 1 out]
        n203 = Divide(x=w346, y=3.3) -> (x/y=w334:dbl)
        "Pitch Roll at Angle" <- w334
        n204 = Multiply(x=w334, y=1.0) -> (x*y=w333:dbl)
        n205 = call <vilib>:"Rotate Z-axis.vi"("error in (no error)"=w498, "angle"=w333, "Scene Object In"=w501) -> ("error out"=w490:errorcluster, "Scene Object Out"=w497:refnum<vi>)  [unwired: 7 in]
        n206 = Merge Errors(w493, w492, w491, w482, w490) -> (w489:errorcluster)
        n207 = Compound Arithmetic op=OR(w489, "STOP", w342) -> (w488:bool)
        n208 = Fract/Exp String To Number(string=w438) -> (number=→"Pitch Closure at Angle":dbl)  [unwired: 3 in, 1 out]
        n209 = Match Pattern(string=w422, regular expression="l") -> (before substring=w439:string)  [unwired: 1 in, 3 out]
        n210 = Divide(x=w344, y=3.194) -> (x/y=→"B Error":dbl)
        n211 = Fract/Exp String To Number(string=w439) -> (number=→"A Error":dbl)  [unwired: 3 in, 1 out]
        "Position Palettes" <- "Motors Absolute Position" ("String")
        "Error Palettes" <- "Error In Motor's Position (in pulses)" ("String")
        "Serial Palettes" <- "No. of Bytes in Serial Comm." ("Serial Palettes")
        "Input Palettes" <- "Input Angles and Speed" ("Input Palettes")
      }
    }
  }
  n212 = Close Reference(reference=w13, error in (no error)=w12) -> (error out=w17:errorcluster)
  n213 = Close Reference(reference=w11, error in (no error)=w17) -> (error out=w16:errorcluster)
  n214 = Close Reference(reference=w10, error in (no error)=w16) -> (error out=w15:errorcluster)
  n215 = VISA Close(VISA resource name=w1, error in (no error)=w2) -> ()  [unwired: 1 out]
  n216 = Close Reference(reference=w9, error in (no error)=w15) -> (error out=w14:errorcluster)
  n217 = Close Reference(reference=w8, error in (no error)=w14) -> (error out=w7:errorcluster)
  n218 = Close Reference(reference=w6, error in (no error)=w7) -> (error out=w5:errorcluster)
  n219 = call <vilib>:"Simple Error Handler.vi"("error in (no error)"=w5) -> ()  [unwired: 4 in, 5 out]
